vi "Multiresolution Analysis - 1D Signal.vi"() -> ()   [LabVIEW 2023]
doc: "This example shows how to use the Multiresolution Analysis Express VI to perform the discrete wavelet transform (DWT)-based multiresolution analysis. You can observe the signal with different resolutions. A large level corresponds to coarse resolution. In addition, you can find that the high-resolution approximation contains all the information of coarse resolution. For example, the approximation at level 2 is the summation of the approximation and the detail at level 3.\n\n<b>Instructions:</b>\nRun this VI. Observe the result of multiresolution analysis."
uses:
  Instance           2 32Saved   Multiresolution Analysis .vi
  Instance           3 32Saved   Multiresolution Analysis .vi
  Instance           4 32Saved   Multiresolution Analysis .vi
  Instance           5 32Saved   Multiresolution Analysis .vi
  Instance           6 32Saved   Multiresolution Analysis .vi
  Instance           7 32Saved   Multiresolution Analysis .vi
panel:
  out "Detail (Level=3)":waveform(dbl)(graph)
  out "Detail (Level=2)":waveform(dbl)(graph)
  out "Detail (Level=1)":waveform(dbl)(graph)
  out "Approximation (Level = 3)":waveform(dbl)(graph)
  out "Approximation (Level = 2)":waveform(dbl)(graph)
  out "Approximation (Level = 1)":waveform(dbl)(graph)
  in  "stop":bool
  out "Signal":waveform(dbl)(graph)
  # "Overview: Shows how to use the Multiresolution Analysis Express VI to perform the discrete wavelet transform (DWT)-based multiresolution analysis.\nRequirements: LabVIEW Full Development System, Advanced Signal Processing Toolkit\nInstructions: \n1. Run this VI. Observe the result of multiresolution analysis.\n2. Click Stop to stop the VI."
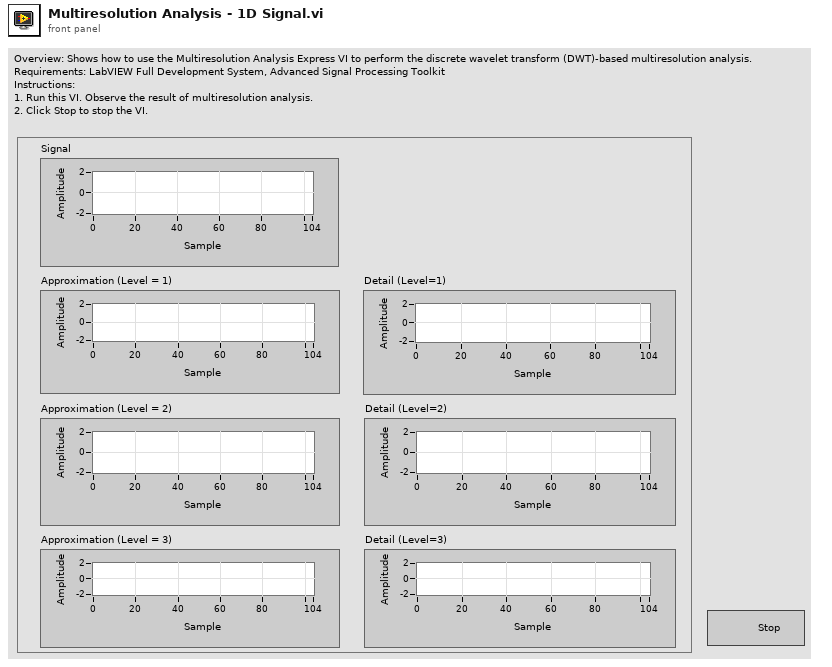
[diagram p1: front panel]
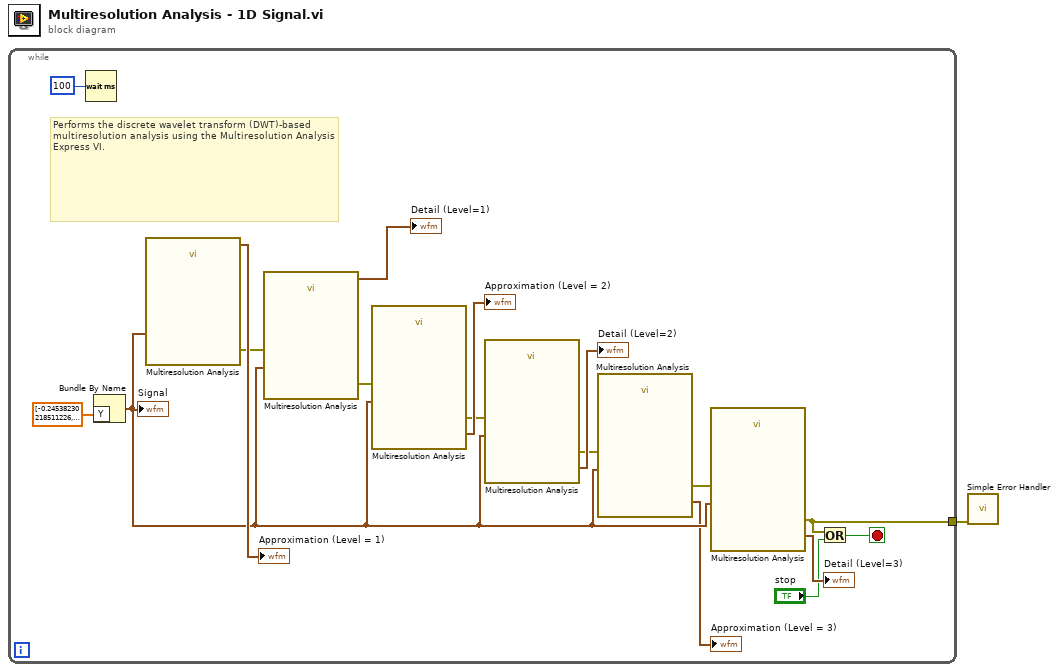
[diagram p0: block diagram]
diagram:
  n1 = while {
    tunnel: [w3] -> w1
    stop <- w5 stop-if-true
    # "Performs the discrete wavelet transform (DWT)-based multiresolution analysis using the Multiresolution Analysis Express VI."
    n2 = Wait (ms)(milliseconds to wait=u32 100) -> ()  [unwired: 1 out]
    n3 = Bundle By Name("Y"=dbl[] [-0.24538230218511226, -0.3060483373063918, -0.3589667545616013, 0.10390613827935703, 0.0963425671535308, 0.08028661776236987, 0.07842272256851149, 0.07463612831538285, 0.09147413377765351, 0.15486095203727077, 0.2175518679677936, 0.2871630414606423, 0.35188795894953767, 0.400075810550012, 0.45363526437227464, 0.5001122456072998, 0.5564051116625117, 0.6450508164063847, 0.7277180626702608, 0.7964186307210345, 0.8626167433759327, 0.936757249334714, 0.997251390508601, 1.8998725574566668, 1.4559988359190448, 0.8098931717474743, 0.24338134141774648, -0.053325035268861766, 0.03657861272580998, 0.4844914609725661, 1.0751121347580395, 1.5959231008008574, 1.811293121408582, 1.7125860758841875, 1.1231808586171719, 0.5531853430059465, 0.48074794842688107, 0.5518151802525989, 0.64125322700255, 0.7197927073978168, 0.8305651570797994, 1.017740674982153, 1.1977184743837281, 1.1691320696207108, 1.0356676685101371, 0.8205915307121884, 0.633219539144189, 0.41917627188351436, 0.2538724172115425, 0.24491832771105876, 0.21800245388324546, 0.10609258256971235, 0.008593154115220908, 0.02291711479694459, -0.03974132473495647, 0.008865426978517827, 0.17731589615203494, 0.028788722172891922, -0.10252039353613529, -0.16711474811809254, -0.23745459185659384, -0.3839582361390131, -0.4683299013587863, -0.5720940964175559, -0.5796811276316892, -0.3445950013674905, -0.9172711335304201, 0.16094122264449762, -0.31801951603558504, -1.2826969990763426, -1.753595568235657, -0.6567217068754156, -0.379290388218691, -1.2437385962665402, -0.284710055701798, -1.122151729065001, -0.9252753753475457, -0.7633885578945547, -1.6199452772876173, -0.6638428473253891, -1.4950179317083532, -0.8972967554385755, -0.8626526257675728, -0.8624341432186192, -0.8504132981502018, -0.7816980689826476, -0.7441725844924705, -0.6858101157472662, -0.680227404771267, -0.8206591146658336, -0.9475571060400942, -1.5978240711861267, -1.3161875243533256, -1.0464963115992014, -0.7520483380662306, -0.4565493834140032, -0.1266961759256651, 0.2777627512595635, -0.6892908908482777, -0.5665886878664512, -0.4447408042943003, -0.3280318819894662, -0.2093248369039546, -0.09362284036854014, 0.02513949594846388] ("Detail (level=3) 2")) -> (w13:waveform(dbl))  [unwired: 1 out]
    "Signal" <- w13
    n4 = call "Multiresolution Analysis"("Signal"=w13) -> ("error out"=w10:errorcluster, "Reconstruction"=→"Approximation (Level = 1)":waveform(dbl))  [unwired: 1 in, 8 out]
    n5 = call "Multiresolution Analysis"("error in (no error)"=w10, "Signal"=w13) -> ("error out"=w9:errorcluster, "Reconstruction"=→"Detail (Level=1)":waveform(dbl))  [unwired: 8 out]
    n6 = call "Multiresolution Analysis"("error in (no error)"=w9, "Signal"=w13) -> ("error out"=w4:errorcluster, "Reconstruction"=→"Approximation (Level = 2)":waveform(dbl))  [unwired: 8 out]
    n7 = call "Multiresolution Analysis"("error in (no error)"=w4, "Signal"=w13) -> ("error out"=w8:errorcluster, "Reconstruction"=→"Detail (Level=2)":waveform(dbl))  [unwired: 8 out]
    n8 = call "Multiresolution Analysis"("error in (no error)"=w8, "Signal"=w13) -> ("error out"=w7:errorcluster, "Reconstruction"=→"Approximation (Level = 3)":waveform(dbl))  [unwired: 8 out]
    n9 = call "Multiresolution Analysis"("error in (no error)"=w7, "Signal"=w13) -> ("error out"=w3:errorcluster, "Reconstruction"=→"Detail (Level=3)":waveform(dbl))  [unwired: 8 out]
    n10 = Or(x=w3, y="stop") -> (x .or. y?=w5:bool)
  }
  n11 = call <vilib>:"Simple Error Handler.vi"("error in (no error)"=w1) -> ()  [unwired: 1 in, 8 out]
